vi "DQMH-GenNet Set Message Blacklist.vi"(7 "Add (T)":bool=TRUE, 8 "error in (no error)":errorcluster, 10 "Message Blacklist":string[](array[string]), 11 "DQMH-GenNet Message Queue in":refnum<class "DQMH-GenNet Message Queue.lvclass">) -> (0 "error out":errorcluster, 3 "DQMH-GenNet Message Queue out":refnum<class "DQMH-GenNet Message Queue.lvclass">)   [LabVIEW 2022 SP3, in "hse-gennet.lvlib" / "DQMH-GenNet Message Queue.lvclass"]
doc: "sets the message message blacklist to the GenNet Message Queue. In default, Add is set to true and the current Blacklist will be extended. If it is set to false, the current Blacklist will be replaced.\n\n____\nHAMPEL SOFTWARE ENGINEERING v3.8.0 (2023-12-18 14:41)"
uses:
  DQMH-GenNet Message Queue.lvclass
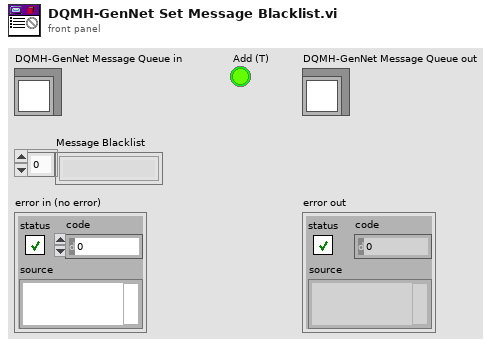
[diagram p1: front panel]
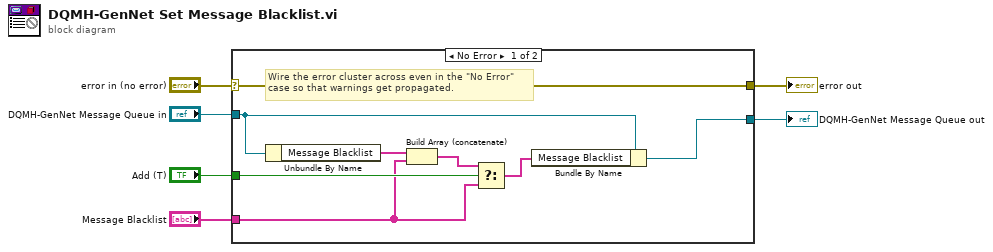
[diagram p0: block diagram]
diagram:
  n1 = case shown="No Error" "error in (no error)" {
    selector: "error in (no error)" -> [w14 w16]
    tunnel: [w14 w16] -> w5
    tunnel: [w13 w15] -> w3
    tunnel: "DQMH-GenNet Message Queue in" -> [w10 w15]
    tunnel: "Add (T)" -> [w12 _]
    tunnel: "Message Blacklist" -> [w8 _]
    frame No Error {
      # "Wire the error cluster across even in the \"No Error\"\ncase so that warnings get propagated."
      n2 = Unbundle By Name(w10) -> ("Message Blacklist"=w9:string[])
      n3 = Build Array (concatenate)(w9, w8) -> (w7:string[])
      n4 = Select(t=w7, s=w12, f=w8) -> (s? t:f=w11:string[])
      n5 = Bundle By Name(cluster=w10, "Message Blacklist"=w11) -> (w13:refnum<class "DQMH-GenNet Message Queue.lvclass">)
    }
    frame Error {
    }
  }
  "error out" <- w5
  "DQMH-GenNet Message Queue out" <- w3
